vi "Get Cluster Control Information OpenG 8.0.vi"(3 "Variant":variant) -> (0 "Name":string[](array[string]), 1 "Data Type":T1[](array[typedef]))   [LabVIEW 2013]
uses:
  <vilib>/Utility/VariantDataType/Type.ctl
  <vilib>/Utility/VariantDataType/VariantType.lvlib
panel:
  out "Error Out":errorcluster
  in  "Error In":errorcluster
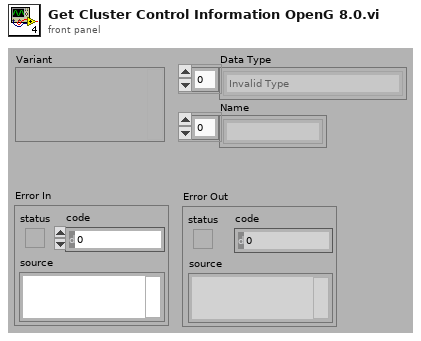
[diagram p1: front panel]
types:
  T1 = typedef "VariantType.lvlib/Type.ctl" = enum8{"Invalid Type", "Void", "I8", "I16", "I32", "I64", "U8", "U16", "U32", "U64", "Single Float", "Double Float", "Extended Float", "Single Complex", "Double Complex", "Extended Complex", "Enum U8", "Enum U16", "Enum U32", "Enum U64", "Single Float With Unit", "Double Float With Unit", "Extended Float With Unit", "Single Complex with Unit", "Double Complex with Unit", "Extended Complex with Unit", "Boolean", "String", "Path", "Picture", "Tag", "Array", "Cluster", "Variant", "LV Variant", "Waveform", "Timestamp", "Digital Waveform", "Digital Data", "ExpressData", "Refnum", "External Data", "VI", "Poly VI", "LabVIEW Class Instance", "Fixed Point"}
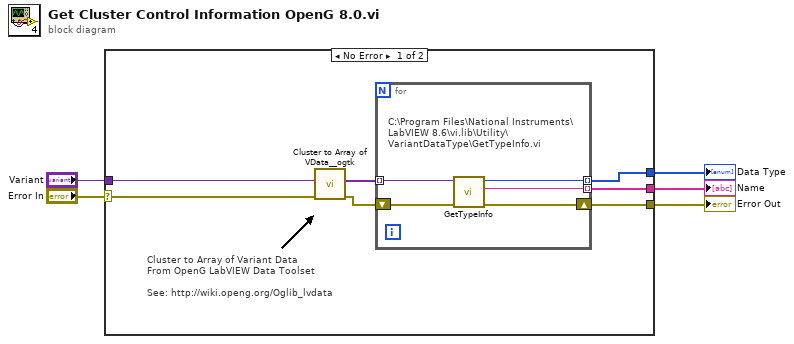
[diagram p0: block diagram]
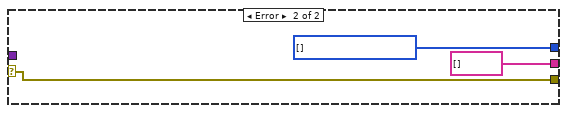
[diagram p2: hidden frame]
diagram:
  n1 = case shown="No Error" "Error In" {
    selector: "Error In" -> [w7 w20]
    tunnel: "Variant" -> [w6 _]
    tunnel: [w10 w20] -> w4
    tunnel: [w9 w19] -> w3
    tunnel: [w8 string[] []] -> w2
    frame No Error {
      # "Cluster to Array of Variant Data\nFrom OpenG LabVIEW Data Toolset \n\nSee: http://wiki.openg.org/Oglib_lvdata"
      n2 = call <userlib>:"Cluster to Array of VData__ogtk.vi"("error in (no error)"=w7, "Cluster"=w6) -> ("error out"=w11:errorcluster, "Array of VData"=w12:variant[])  [unwired: 8 out]
      n3 = for {
        tunnel: w12 -> [w17] mode=indexing
        shift-right: [w15] -> w10
        shift-left: w11 -> [w16]
        tunnel: [w14] -> w9 mode=indexing
        tunnel: [w13] -> w8 mode=indexing
        # "C:\\Program Files\\National Instruments\\LabVIEW 8.6\\vi.lib\\Utility\\VariantDataType\\GetTypeInfo.vi"
        n4 = call <vilib>:"GetTypeInfo.vi"("error in (no error)"=w16, "Variant"=w17) -> ("error out"=w15:errorcluster, "Name"=w13:string, "Type Enum"=w14:T1)  [unwired: 7 out]
      }
    }
    frame Error {
      w19 = T1[] [] items=["Invalid Type", "Void", "I8", "I16", "I32", "I64", "U8", "U16", "U32", "U64", "Single Float", "Double Float", "Extended Float", "Single Complex", "Double Complex", "Extended Complex", "Enum U8", "Enum U16", "Enum U32", "Enum U64", "Single Float With Unit", "Double Float With Unit", "Extended Float With Unit", "Single Complex with Unit", "Double Complex with Unit", "Extended Complex with Unit", "Boolean", "String", "Path", "Picture", "Tag", "Array", "Cluster", "Variant", "LV Variant", "Waveform", "Timestamp", "Digital Waveform", "Digital Data", "ExpressData", "Refnum", "External Data", "VI", "Poly VI", "LabVIEW Class Instance", "Fixed Point"]
    }
  }
  "Error Out" <- w4
  "Data Type" <- w3
  "Name" <- w2
